vi "writesettings.vi"(0 "COEFFICIENT":T1, 2 "Tangent":T2, 9 "BLUE":T3, 11 "RED":T3) -> ()   [LabVIEW 2012]
uses:
  <vilib>/Utility/config.llb/NI_LVConfig.lvlib
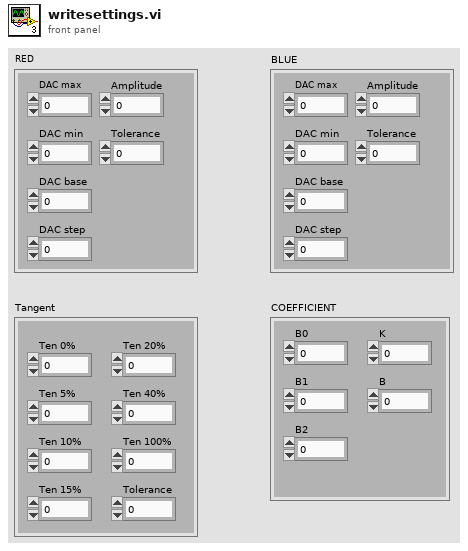
[diagram p1: front panel]
types:
  T1 = cluster{"B0":dbl, "B1":dbl, "K":dbl, "B":dbl, "B2":dbl}
  T2 = cluster{"Ten 0%":dbl, "Ten 5%":dbl, "Ten 10%":dbl, "Ten 20%":dbl, "Tolerance":dbl, "Ten 15%":dbl, "Ten 40%":dbl, "Ten 100%":dbl}
  T3 = cluster{"DAC max":dbl, "DAC min":dbl, "DAC base":dbl, "DAC step":dbl, "Amplitude":dbl, "Tolerance":dbl}
  T4 = cluster{"Ten 0%":dbl, "Ten 5%":dbl, "Ten 10%":dbl, "Ten 15%":dbl, "Tolerance":dbl, "Ten 20%":dbl, "Ten 40%":dbl, "Ten 100%":dbl}
  T5 = cluster{"B0":dbl, "B1":dbl, "B2":dbl, "K":dbl, "B":dbl}
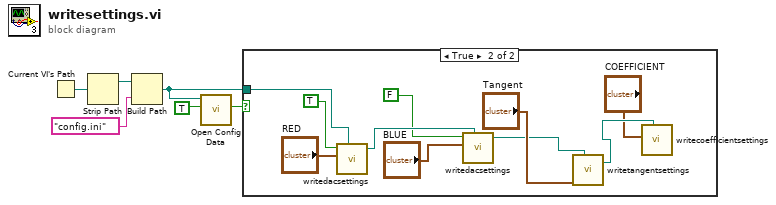
[diagram p0: block diagram]
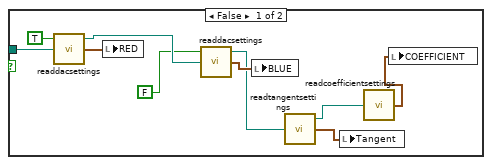
[diagram p2: hidden frame]
diagram:
  n1 = Current VI's Path() -> (path=w1:path)
  n2 = Strip Path(path=w1) -> (stripped path=w2:path)  [unwired: 1 out]
  n3 = Build Path(base path=w2, name or relative path="config.ini") -> (appended path=w3:path)
  n4 = call <vilib>:"Open Config Data.vi"("create file if necessary (T)"=TRUE, "configuration file path"=w3) -> ("file created?"=w4:bool)  [unwired: 7 in, 2 out]
  n5 = case shown="True" w4 {
    tunnel: w3 -> [w15 w25]
    frame False {
      n6 = call "readdacsettings.vi"("red"=TRUE, "Path"=w15) -> ("Path 2"=w13:path, 6:w14:T3)  [unwired: 3 in, 1 out]
      n7 = local write "RED"(w14) -> ()
      n8 = call "readdacsettings.vi"("red"=FALSE, "Path"=w13) -> ("Path 2"=w8:path, 6:w11:T3)  [unwired: 3 in, 1 out]
      n9 = local write "BLUE"(w11) -> ()
      n10 = call "readtangentsettings.vi"("Path"=w8) -> ("Path 2"=w10:path, 6:w9:T4)  [unwired: 4 in, 1 out]
      n11 = local write "Tangent"(w9) -> ()
      n12 = call "readcoefficientsettings.vi"("Path"=w10) -> (6:w7:T5)  [unwired: 4 in, 2 out]
      n13 = local write "COEFFICIENT"(w7) -> ()
    }
    frame True {
      n14 = call "writedacsettings.vi"("red"=TRUE, "Path"=w25, 2:"RED") -> ("Path 2"=w23:path)  [unwired: 4 in, 1 out]
      n15 = call "writedacsettings.vi"("red"=FALSE, "Path"=w23, 2:"BLUE") -> ("Path 2"=w19:path)  [unwired: 4 in, 1 out]
      n16 = call "writetangentsettings.vi"("Path"=w19, 4:"Tangent") -> ("Path 2"=w18:path)  [unwired: 4 in, 1 out]
      n17 = call "writecoefficientsettings.vi"("Path"=w18, 2:"COEFFICIENT") -> ()  [unwired: 5 in, 2 out]
    }
  }
